vi "Match End.vi"(8 "error in (no error)":errorcluster, 11 "Alpaca Parser in":refnum<class "Parser.lvclass">) -> (0 "error out":errorcluster, 3 "Alpaca Parser out":refnum<class "Parser.lvclass">)   [LabVIEW 2013, in "JKI JSON Serialization.lvlib" / "Parser.lvclass"]
uses:
  Parser.lvclass
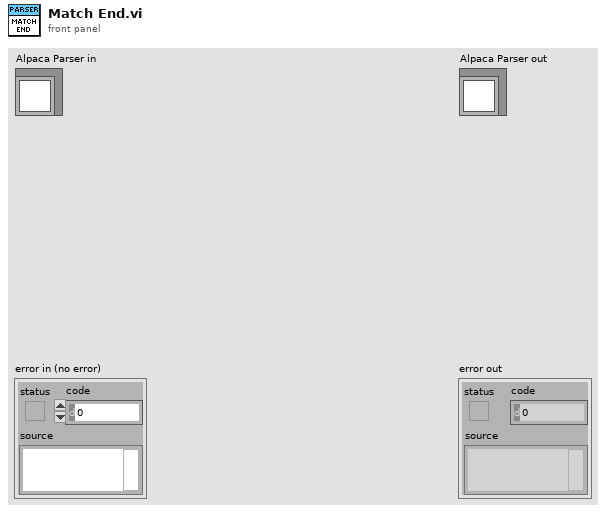
[diagram p1: front panel]
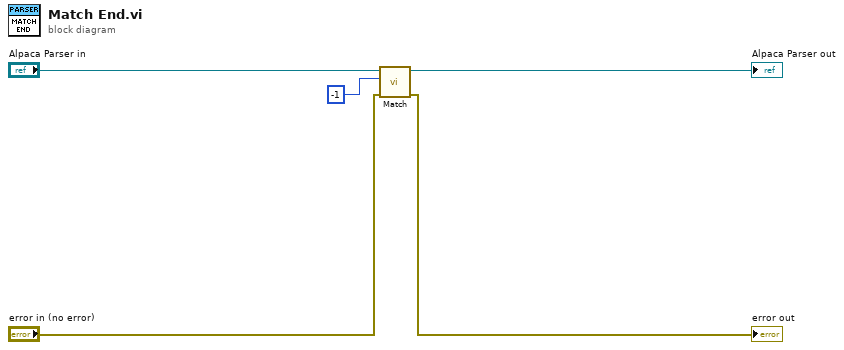
[diagram p0: block diagram]
diagram:
  n1 = call-dynamic "Match.vi"("error in (no error)"="error in (no error)", "Token Type"=-1, "Alpaca Parser in"="Alpaca Parser in") -> ("error out"=→"error out":errorcluster, "Alpaca Parser out"=→"Alpaca Parser out":refnum<class "Parser.lvclass">)  [unwired: 7 in]
